vi "retrieveTable--double.vi"(8 "error in (no error)":errorcluster, 11 "MS-Excel in":refnum<class "MS-Excel.lvclass">) -> (0 "error out":errorcluster, 2 "Table":dbl[][](array[numeric]), 3 "MS-Excel out":refnum<class "MS-Excel.lvclass">)   [LabVIEW 2017, in "LabVIEW NPOI.lvlib" / "MS-Excel.lvclass"]
doc: "Protected dynamic dispatch method to append the wire <b>Table</b> as 2D array of strings to the <b>Document</b> as a table."
uses:
  MS-Excel.lvclass
  C:/Users/Neo/Desktop/Dev_Tools_BR/LabVIEW_NPOI/lib/NPOI 2.1.1/NPOI.dll
  lib/NPOI 2.1.1/NPOI.dll
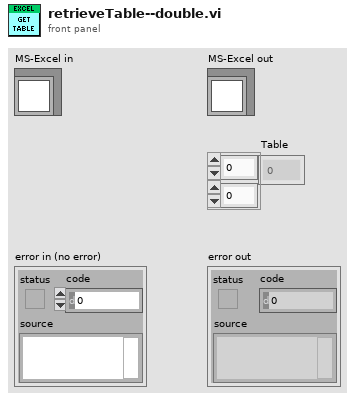
[diagram p1: front panel]
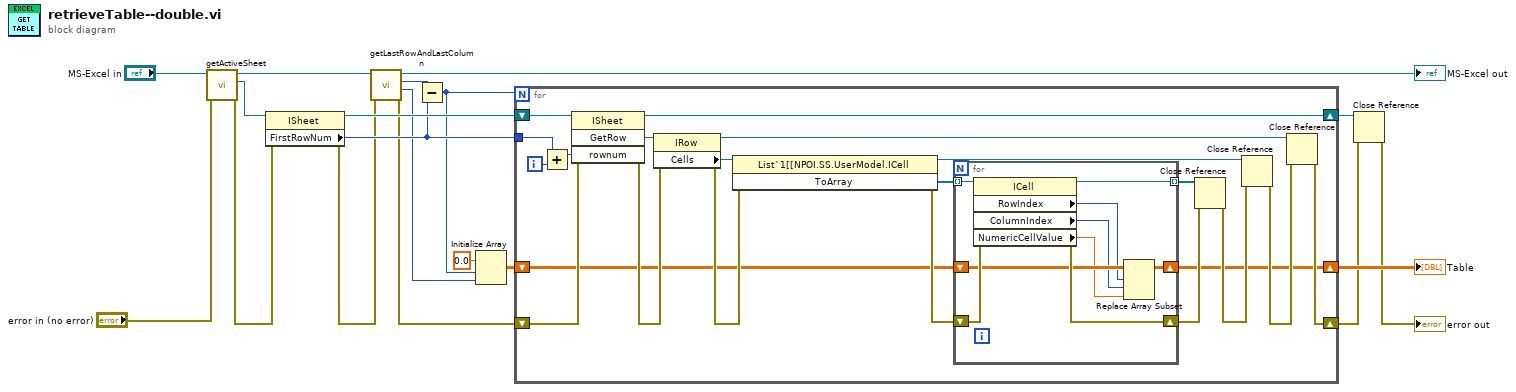
[diagram p0: block diagram]
diagram:
  n1 = call-dynamic "getActiveSheet.vi"("error in (no error)"="error in (no error)", "MS-Excel in"="MS-Excel in") -> ("error out"=w15:errorcluster, "Sheet Ref"=w17:refnum<k24>, "MS-Excel out"=w18:refnum<class "MS-Excel.lvclass">)  [unwired: 6 in, 1 out]
  n2 = property class="ISheet"(reference=w17, error in=w15) -> (reference out=w16:refnum<k24>, error out=w5:errorcluster, "FirstRowNum"=w13:i32)
  n3 = call-dynamic "getLastRowAndLastColumn.vi"("error in (no error)"=w5, "MS-Excel in"=w18) -> ("error out"=w4:errorcluster, "Last Column"=w7:i32, "Last Row"=w11:i32, "MS-Excel out"=→"MS-Excel out":refnum<class "MS-Excel.lvclass">)  [unwired: 6 in]
  n4 = Subtract(x=w11, y=w13) -> (x-y=w8:i32)
  n5 = Initialize Array(0.0, w8, w7) -> (w6:dbl[][])
  n6 = for {
    N: w8 -> [_]
    shift-right: [w28] -> w2
    shift-left: w4 -> [w35]
    tunnel: w13 -> [w32]
    shift-right: [w29] -> w3
    shift-left: w16 -> [w40]
    shift-right: [w21] -> w10
    shift-left: w6 -> [w22]
    i -> [w30]
    n7 = Add(x=w32, y=w30) -> (x+y=w31:i32)
    n8 = invoke class="ISheet" method="GetRow"(reference=w40, error in=w35, "rownum"=w31) -> (reference out=w29:refnum<k24>, error out=w34:errorcluster, "GetRow"=w39:refnum<k24>)  [unwired: 1 in, 1 out]
    n9 = property class="IRow"(reference=w39, error in=w34) -> (reference out=w36:refnum<k24>, error out=w33:errorcluster, "Cells"=w20:refnum<k24>)
    n10 = invoke class="List`1[[NPOI.SS.UserModel.ICell" method="ToArray"(reference=w20, error in=w33) -> (reference out=w38:refnum<k24>, error out=w27:errorcluster, "ToArray"=w26:refnum<k24>[])  [unwired: 1 in]
    n11 = for {
      tunnel: w26 -> [w49] mode=indexing
      shift-right: [w46] -> w24
      shift-left: w27 -> [w48]
      tunnel: [w47] -> w25 mode=indexing
      shift-right: [w44] -> w21
      shift-left: w22 -> [w45]
      n12 = property class="ICell"(reference=w49, error in=w48) -> (reference out=w47:refnum<k24>, error out=w46:errorcluster, "RowIndex"=w43:i32, "ColumnIndex"=w42:i32, "NumericCellValue"=w41:dbl)
      n13 = Replace Array Subset(array=w45, new element=w41, index (row)=w43, index (col)=w42) -> (w44:dbl[][])
    }
    n14 = Close Reference(reference=w25, error in (no error)=w24) -> (error out=w23:errorcluster)
    n15 = Close Reference(reference=w38, error in (no error)=w23) -> (error out=w37:errorcluster)
    n16 = Close Reference(reference=w36, error in (no error)=w37) -> (error out=w28:errorcluster)
  }
  "Table" <- w10
  n17 = Close Reference(reference=w3, error in (no error)=w2) -> (error out=→"error out":errorcluster)
